vi "Read.vi"(8 "error in (no error)":errorcluster, 9 "Command To Write":string, 10 "Bytes to Read (11)":u32=11, 11 "VISA resource name":refnum<visa-resource-name>) -> (0 "error out":errorcluster, 2 "Ultimus V Feedback Data":string, 3 "VISA resource name out":refnum<visa-resource-name>)   [LabVIEW 2016, in "EFD Ultimus V.lvlib"]
doc: "Reads data from the Ultimus V unit. Bytes to read sets the read buffer size."
uses:
  EFD Ultimus V.lvlib
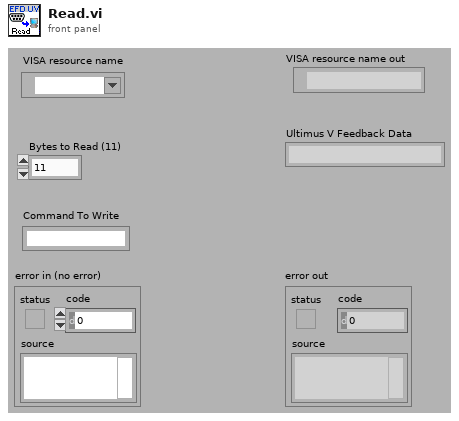
[diagram p1: front panel]
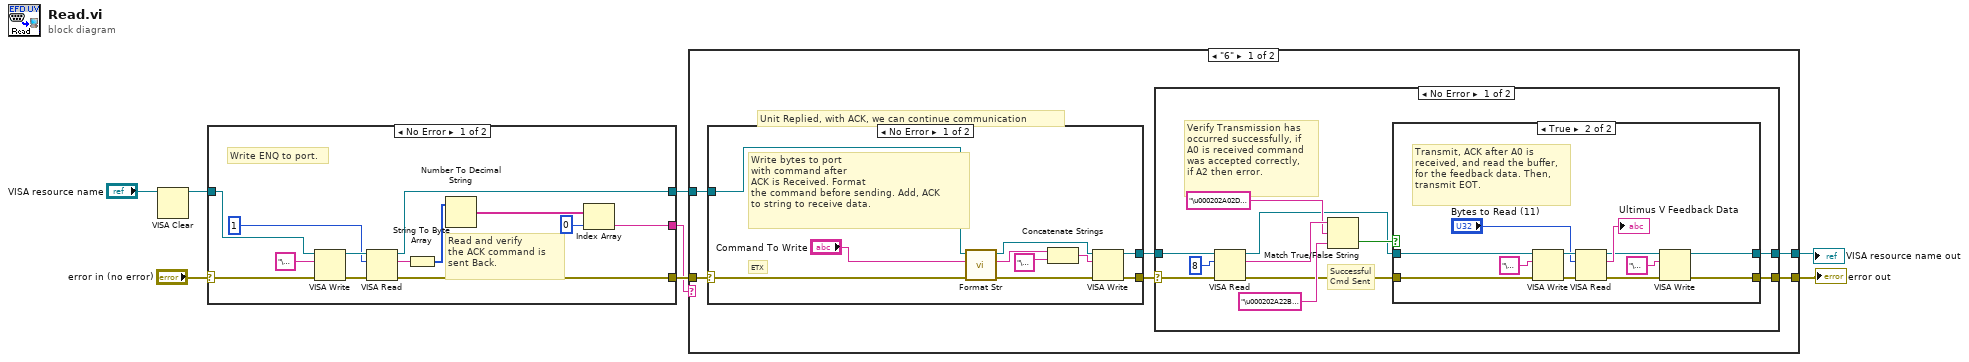
[diagram p0: block diagram]
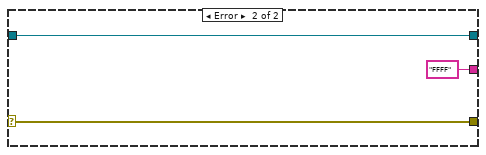
[diagram p2: hidden frame]
diagram:
  n1 = VISA Clear(VISA resource name="VISA resource name") -> (VISA resource name out=w7:refnum<visa-resource-name>)  [unwired: 1 in, 1 out]
  n2 = case shown="No Error" "error in (no error)" {
    selector: "error in (no error)" -> [w21 w24]
    tunnel: [w15 w23] -> w6
    tunnel: [w16 w24] -> w5
    tunnel: w7 -> [w20 w23]
    tunnel: [w10 "FFFF" ("read buffer")] -> w4
    frame No Error {
      # "Read and verify \nthe ACK command is \nsent Back."
      # "Write ENQ to port."
      n3 = VISA Write(VISA resource name=w20, write buffer="\u0005", error in (no error)=w21) -> (VISA resource name out=w18:refnum<visa-resource-name>, error out=w17:errorcluster)  [unwired: 1 out]
      n4 = VISA Read(VISA resource name=w18, byte count=u32 1, error in (no error)=w17) -> (VISA resource name out=w15:refnum<visa-resource-name>, read buffer=w14:string, error out=w16:errorcluster)  [unwired: 1 out]
      n5 = String To Byte Array(string=w14) -> (unsigned byte array=w13:u8[])
      n6 = Number To Decimal String(number=w13) -> (decimal integer string=w12:string[])  [unwired: 1 out]
      n7 = Index Array(array=w12, index=0) -> (element=w10:string)
    }
    frame Error {
    }
  }
  n8 = case shown="\"6\"" w4 {
    tunnel: [w26 w71] -> w3
    tunnel: w6 -> [w28 w71]
    tunnel: w5 -> [w27 w70]
    tunnel: [w25 w70] -> w1
    frame "6" {
      # "Unit Replied, with ACK, we can continue communication"
      n9 = case shown="No Error" w27 {
        selector: w27 -> [w63 w69]
        tunnel: [w66 w68] -> w30
        tunnel: [w67 w69] -> w29
        tunnel: w28 -> [w58 w68]
        frame No Error {
          # "ETX"
          # "Write bytes to port\nwith command after\nACK is Received. Format \nthe command before sending. Add, ACK \nto string to receive data."
          n10 = call "Format Str.vi"("error in (no error)"=w63, "Input Cmd String"="Command To Write", "VISA resource name"=w58) -> ("error out"=w62:errorcluster, "Formatted Cmd String"=w60:string, "VISA resource name out"=w59:refnum<visa-resource-name>)  [unwired: 6 in]
          n11 = Concatenate Strings(w60, "\u0006" ("string")) -> (w65:string)
          n12 = VISA Write(VISA resource name=w59, write buffer=w65, error in (no error)=w62) -> (VISA resource name out=w66:refnum<visa-resource-name>, error out=w67:errorcluster)  [unwired: 1 out]
        }
        frame Error {
        }
      }
      n13 = case "Read bytes from port." shown="No Error" w29 {
        selector: w29 -> [w40 w56]
        tunnel: [w31 w56] -> w25
        tunnel: [w33 w57] -> w26
        tunnel: w30 -> [w41 w57]
        frame No Error {
          # "Verify Transmission has\noccurred successfully, if\nA0 is received command\nwas accepted correctly,\nif A2 then error."
          # "Successful \nCmd Sent"
          n14 = VISA Read(VISA resource name=w41, byte count=u32 8, error in (no error)=w40) -> (VISA resource name out=w34:refnum<visa-resource-name>, read buffer=w39:string, error out=w32:errorcluster)  [unwired: 1 out]
          n15 = Match True/False String(2:"\u000202A22B\u0003" ("false string"), 3:"\u000202A02D\u0003" ("true string"), 4:w39) -> (0:w35:bool)  [unwired: 1 out]
          n16 = case shown="True" w35 {
            tunnel: w34 -> [w43 w55]
            tunnel: [w43 w46] -> w33
            tunnel: w32 -> [w42 w54]
            tunnel: [w42 w48] -> w31
            frame False {
            }
            frame True {
              # "Transmit, ACK after A0 is\nreceived, and read the buffer,\nfor the feedback data. Then,\ntransmit EOT."
              n17 = VISA Write(VISA resource name=w55, write buffer="\u0006", error in (no error)=w54) -> (VISA resource name out=w52:refnum<visa-resource-name>, error out=w51:errorcluster)  [unwired: 1 out]
              n18 = VISA Read(VISA resource name=w52, byte count="Bytes to Read (11)", error in (no error)=w51) -> (VISA resource name out=w47:refnum<visa-resource-name>, read buffer=→"Ultimus V Feedback Data":string, error out=w49:errorcluster)  [unwired: 1 out]
              n19 = VISA Write(VISA resource name=w47, write buffer="\u0004", error in (no error)=w49) -> (VISA resource name out=w46:refnum<visa-resource-name>, error out=w48:errorcluster)  [unwired: 1 out]
            }
          }
        }
        frame Error {
          # "Error occurred \nreading Bytes at \nSerial Port"
        }
      }
    }
    frame Default {
      # "Could not communicated with the unit."
    }
  }
  "VISA resource name out" <- w3
  "error out" <- w1
